vi "Publish to Message Subscribers.vi"(8 "error in (no error)":errorcluster, 9 "Message Priority (Normal)":T2, 10 "Message in":refnum<class "Message.lvclass">, 11 "Message Subsciptions in":T1[](array[typedef])) -> (0 "error out":errorcluster, 1 "Callers found?":bool, 3 "Subsciptions out":T1[](array[typedef]))   [LabVIEW 2020, in "Publisher.lvlib" / "Publisher.lvclass"]
doc: "Get enqueuers in the hierarchy of 'Message in' and publish to these. All dead enqueuers are removed without throwing an error."
uses:
  Publisher.lvclass
  PPL/HDH.Actor Framework.Core.Actor.lvlibp/1abvi3w/vi.lib/ActorFramework/Message/Message.lvclass
  PPL/HDH.Actor Framework.Core.Actor.lvlibp/1abvi3w/vi.lib/ActorFramework/Message Enqueuer/Message Priority.ctl
  Controls/Ctl_Subscription Element.ctl
  PPL/HDH.Actor Framework.Core.Actor.lvlibp/1abvi3w/vi.lib/ActorFramework/Message Enqueuer/Message Enqueuer.lvclass
  db873f7a-0b02-498f-8e83-1c0f04c767f7.vi
  PPL/HDH.Actor Framework.Core.Utility.lvlibp
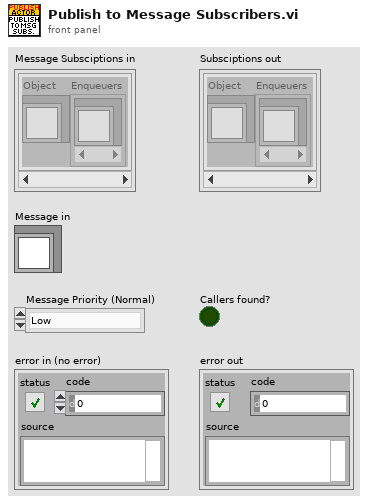
[diagram p1: front panel]
types:
  T1 = typedef "Publisher.lvlib/Publisher.lvclass/Ctl_Subscription Element.ctl" = cluster{"Object":refnum<class>, "Enqueuers":refnum<class "Message Enqueuer.lvclass">[]}
  T2 = typedef "HDH.Actor Framework.Core.Actor.lvlibp/Message Enqueuer.lvclass/Message Priority.ctl" = enum16{"Low", "Normal", "High"}
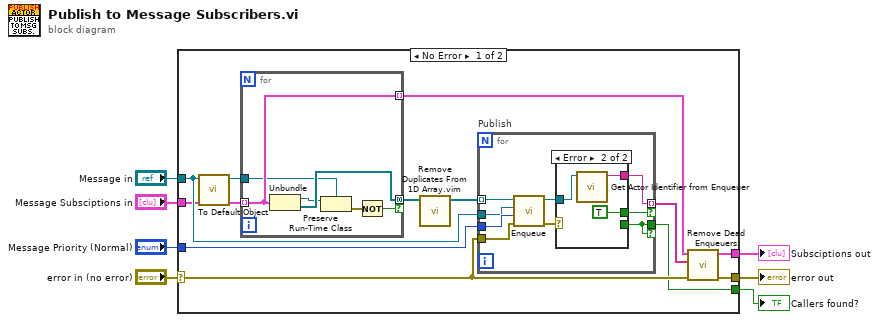
[diagram p0: block diagram]
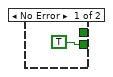
[diagram p2: hidden frame]
diagram:
  n1 = case shown="No Error" "error in (no error)" {
    selector: "error in (no error)" -> [w11 w40]
    tunnel: [w19 w40] -> w7
    tunnel: "Message Priority (Normal)" -> [w18 _]
    tunnel: "Message in" -> [w16 _]
    tunnel: "Message Subsciptions in" -> [w10 w39]
    tunnel: [w12 w39] -> w3
    tunnel: [w8 _] -> w1
    frame No Error {
      n2 = call "To Default Object.vi"("Object in"=w16) -> ("Default out"=w17:refnum<class "Message.lvclass">)  [unwired: 10 in]
      n3 = for {
        tunnel: w17 -> [w20]
        tunnel: w10 -> [w22] mode=indexing
        tunnel: [w24] -> w15 mode=concatenating if=w23
        tunnel: [w22] -> w9 mode=indexing
        n4 = Unbundle(w22) -> ("Object"=w21:refnum<class>, "Enqueuers"=w24:refnum<class "Message Enqueuer.lvclass">[])
        n5 = Preserve Run-Time Class(object in=w21, 2:w20) -> (error out=w25:errorcluster)  [unwired: 1 in, 1 out]
        n6 = Not(x=w25) -> (.not. x?=w23:bool)
      }
      n7 = call "Remove Duplicates From 1D Array.vim"("array"=w15) -> ("array with duplicates removed"=w14:refnum<class "Message Enqueuer.lvclass">[])  [unwired: 10 in]
      n8 = for "Publish" {
        tunnel: w14 -> [w34] mode=indexing
        tunnel: w18 -> [w33]
        tunnel: w16 -> [w32]
        tunnel: [w29] -> w13 mode=indexing if=w28
        tunnel: w11 -> [w27]
        tunnel: [w26] -> w8 if=w26
        n9 = call "Enqueue.vi"("error in (no error)"=w27, "Message Priority (Normal)"=w33, "Message"=w32, "Message Enqueuer in"=w34) -> ("error out"=w31:errorcluster, "Message Enqueuer out"=w30:refnum<class "Message Enqueuer.lvclass">)  [unwired: 6 in]
        n10 = case shown="Error" w31 {
          tunnel: w30 -> [_ w38]
          tunnel: [_ w37] -> w29
          tunnel: [_ TRUE] -> w28
          tunnel: [TRUE _] -> w26
          frame No Error {
          }
          frame Error {
            n11 = call "Get Actor Identifier from Enqueuer.vi"("Message Enqueuer in"=w38) -> ("Actor ID string out"=w37:string)  [unwired: 9 in, 1 out]
          }
        }
      }
      n12 = call "Remove Dead Enqueuers.vi"("error in (no error)"=w11, "Enqueuers to remove"=w13, "Subsciptions in"=w9) -> ("error out"=w19:errorcluster, "Subsciptions out"=w12:T1[])  [unwired: 7 in]
    }
    frame Error {
    }
  }
  "error out" <- w7
  "Subsciptions out" <- w3
  "Callers found?" <- w1
